vi "Example Interruption 1.vi"(8 "Error In":errorcluster) -> (0 "Error Out":errorcluster)   [LabVIEW 2014]
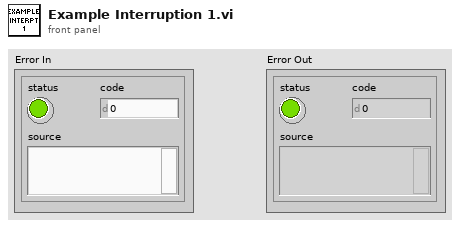
[diagram p1: front panel]
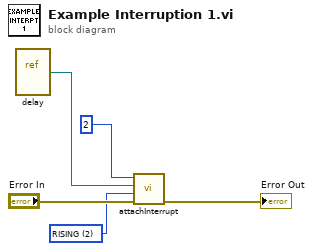
[diagram p0: block diagram]
diagram:
  w2 = u16 2 items=["LOW", "CHANGE", "RISING", "FALLING", "HIGH"] ("mode")
  n1 = vi-ref "delay.vi"() -> (w1:refnum<vi>)
  n2 = call "attachInterrupt.vi"("Error In"="Error In", "mode"=w2, "VI Refnum"=w1, "pin number"=2) -> ("Error Out"=→"Error Out":errorcluster)  [unwired: 7 in]
